vi "repeat cycle_linear up.vi"(8 "error in (no error)":errorcluster caption="에러 입력(에러 없음)", 10 "waveform in":waveform(dbl), 11 "Waveform Obj 입력":refnum<class "PWL_DW7802.lvclass">) -> (0 "error out":errorcluster caption="에러 출력", 2 "waveform out":waveform(dbl), 3 "Waveform Obj 출력":refnum<class "PWL_DW7802.lvclass">)   [LabVIEW 2020, in "PWL_DW7802.lvclass"]
uses:
  PWL_DW7802.lvclass
  Waveform Gen/Waveform Gen.lvclass/Waveform Gen.ctl
  PWL/PWL.lvclass/PWL.ctl
  Waveform Gen/Accessors/Read cycle.vi
  Waveform Gen/Accessors/Read scale.vi
  PWL/Accessors/Read previous pwl scale.vi
  <vilib>/Waveform/WDTOps.llb/WDT Number of Waveform Samples DBL.vi
  <vilib>/Waveform/WDTOps.llb/WDT Get Waveform Subset DBL.vi
  <vilib>/Waveform/WDTOps.llb/WDT Append Waveforms DBL.vi
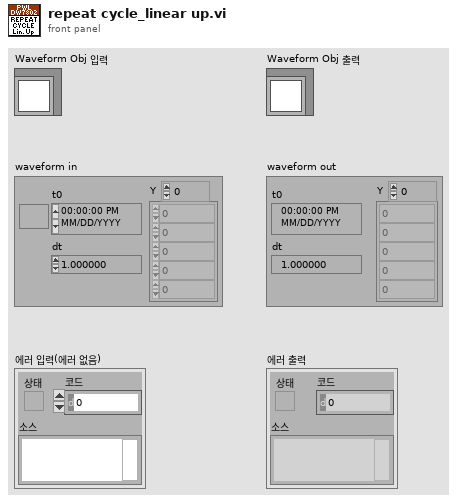
[diagram p1: front panel]
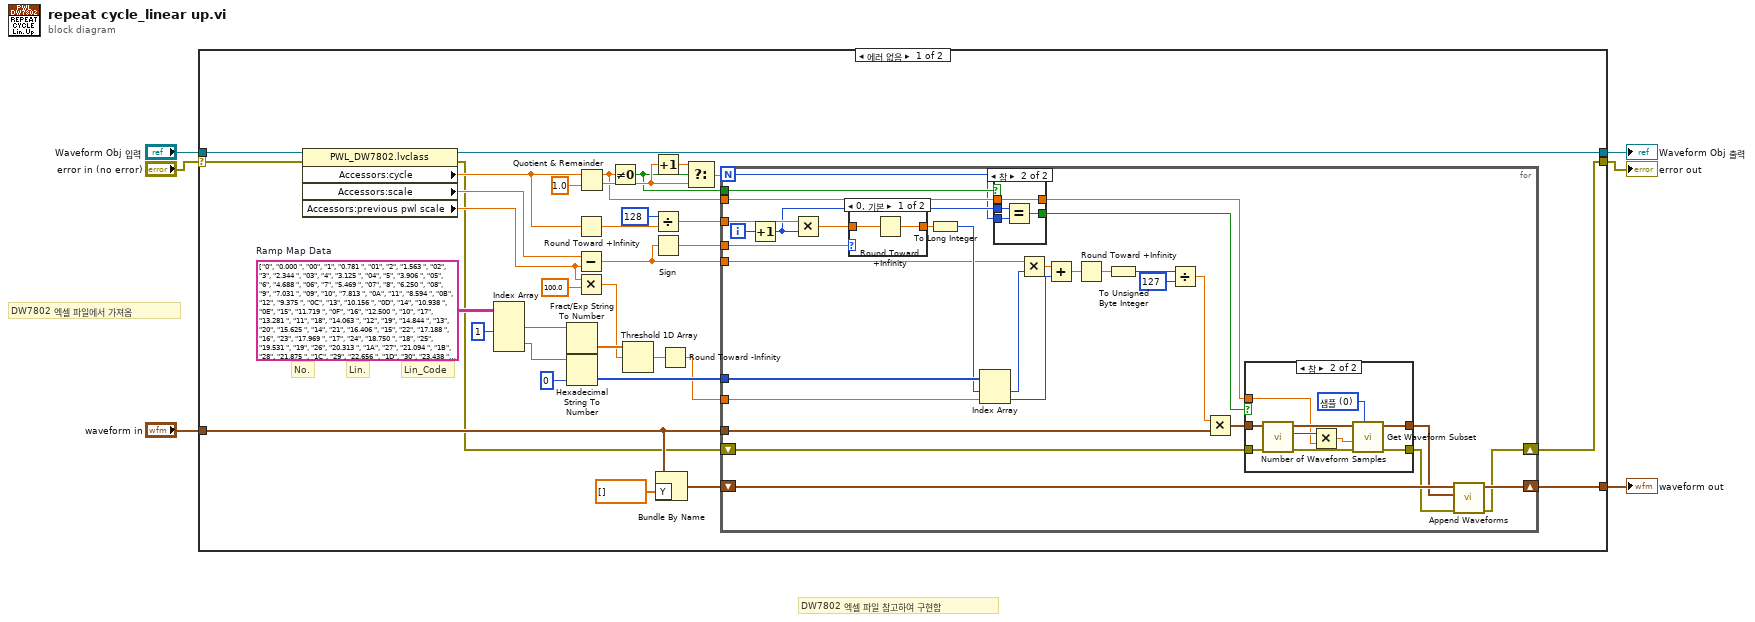
[diagram p0: block diagram]
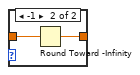
[diagram p2: hidden frame]
diagram:
  # "DW7802 엑셀 파일에서 가져옴"
  # "DW7802 엑셀 파일 참고하여 구현함"
  n1 = case shown="에러 없음" "error in (no error)" {
    selector: "error in (no error)" -> [w39 w92]
    tunnel: "Waveform Obj 입력" -> [w40 w93]
    tunnel: [w38 w93] -> w4
    tunnel: [w15 w92] -> w3
    tunnel: "waveform in" -> [w22 _]
    tunnel: [w14 _] -> w1
    frame No Error {
      w32 = string[][] [["0", "0.000 ", "00"], ["1", "0.781 ", "01"], ["2", "1.563 ", "02"], ["3", "2.344 ", "03"], ["4", "3.125 ", "04"], ["5", "3.906 ", "05"], ["6", "4.688 ", "06"], ["7", "5.469 ", "07"], ["8", "6.250 ", "08"], ["9", "7.031 ", "09"], ["10", "7.813 ", "0A"], ["11", "8.594 ", "0B"], ["12", "9.375 ", "0C"], ["13", "10.156 ", "0D"], ["14", "10.938 ", "0E"], ["15", "11.719 ", "0F"], ["16", "12.500 ", "10"], ["17", "13.281 ", "11"], ["18", "14.063 ", "12"], ["19", "14.844 ", "13"], ["20", "15.625 ", "14"], ["21", "16.406 ", "15"], ["22", "17.188 ", "16"], ["23", "17.969 ", "17"], ["24", "18.750 ", "18"], ["25", "19.531 ", "19"], ["26", "20.313 ", "1A"], ["27", "21.094 ", "1B"], ["28", "21.875 ", "1C"], ["29", "22.656 ", "1D"], ["30", "23.438 ", "1E"], ["31", "24.219 ", "1F"], ["32", "25.000 ", "20"], ["33", "25.781 ", "21"], ["34", "26.563 ", "22"], ["35", "27.344 ", "23"], ["36", "28.125 ", "24"], ["37", "28.906 ", "25"], ["38", "29.688 ", "26"], ["39", "30.469 ", "27"], ["40", "31.250 ", "28"], ["41", "32.031 ", "29"], ["42", "32.813 ", "2A"], ["43", "33.594 ", "2B"], ["44", "34.375 ", "2C"], ["45", "35.156 ", "2D"], ["46", "35.938 ", "2E"], ["47", "36.719 ", "2F"], ["48", "37.500 ", "30"], ["49", "38.281 ", "31"], ["50", "39.063 ", "32"], ["51", "39.844 ", "33"], ["52", "40.625 ", "34"], ["53", "41.406 ", "35"], ["54", "42.188 ", "36"], ["55", "42.969 ", "37"], ["56", "43.750 ", "38"], ["57", "44.531 ", "39"], ["58", "45.313 ", "3A"], ["59", "46.094 ", "3B"], ["60", "46.875 ", "3C"], ["61", "47.656 ", "3D"], ["62", "48.438 ", "3E"], ["63", "49.219 ", "3F"], ["64", "50.000 ", "40"], ["65", "50.781 ", "40"], ["66", "51.563 ", "41"], ["67", "52.344 ", "42"], ["68", "53.125 ", "43"], ["69", "53.906 ", "44"], ["70", "54.688 ", "45"], ["71", "55.469 ", "46"], ["72", "56.250 ", "47"], ["73", "57.031 ", "48"], ["74", "57.813 ", "49"], ["75", "58.594 ", "4A"], ["76", "59.375 ", "4B"], ["77", "60.156 ", "4C"], ["78", "60.938 ", "4D"], ["79", "61.719 ", "4E"], ["80", "62.500 ", "4F"], ["81", "63.281 ", "50"], ["82", "64.063 ", "51"], ["83", "64.844 ", "52"], ["84", "65.625 ", "53"], ["85", "66.406 ", "54"], ["86", "67.188 ", "55"], ["87", "67.969 ", "56"], ["88", "68.750 ", "57"], ["89", "69.531 ", "58"], ["90", "70.313 ", "59"], ["91", "71.094 ", "5A"], ["92", "71.875 ", "5B"], ["93", "72.656 ", "5C"], ["94", "73.438 ", "5D"], ["95", "74.219 ", "5E"], ["96", "75.000 ", "5F"], ["97", "75.781 ", "60"], ["98", "76.563 ", "61"], ["99", "77.344 ", "62"], ["100", "78.125 ", "63"], ["101", "78.906 ", "64"], ["102", "79.688 ", "65"], ["103", "80.469 ", "66"], ["104", "81.250 ", "67"], ["105", "82.031 ", "68"], ["106", "82.813 ", "69"], ["107", "83.594 ", "6A"], ["108", "84.375 ", "6B"], ["109", "85.156 ", "6C"], ["110", "85.938 ", "6D"], ["111", "86.719 ", "6E"], ["112", "87.500 ", "6F"], ["113", "88.281 ", "70"], ["114", "89.063 ", "71"], ["115", "89.844 ", "72"], ["116", "90.625 ", "73"], ["117", "91.406 ", "74"], ["118", "92.188 ", "75"], ["119", "92.969 ", "76"], ["120", "93.750 ", "77"], ["121", "94.531 ", "78"], ["122", "95.313 ", "79"], ["123", "96.094 ", "7A"], ["124", "96.875 ", "7B"], ["125", "97.656 ", "7C"], ["126", "98.438 ", "7D"], ["127", "99.219 ", "7E"], ["128", "100.000 ", "7F"]]  # Ramp Map Data
      # "Lin_Code"
      # "Lin."
      # "No."
      n2 = property class="PWL_DW7802.lvclass"(reference=w40, error in=w39) -> (reference out=w38:refnum<class "PWL_DW7802.lvclass">, error out=w16:errorcluster, "Accessors:cycle"=w26:dbl, "Accessors:scale"=w29:dbl, "Accessors:previous pwl scale"=w28:dbl)
      n3 = Index Array(array=w32, index (col) #1=1 ("비활성화된 인덱스 (열)")) -> (element #1=w37:string[], element #2=w30:string[])  [unwired: 3 in]
      n4 = Fract/Exp String To Number(string=w37) -> (number=w11:dbl[])  [unwired: 3 in, 1 out]
      n5 = Hexadecimal String To Number(string=w30, default (0uL)=u8 0) -> (number=w36:u8[])  [unwired: 1 in, 1 out]
      n6 = Round Toward +Infinity(x=w26) -> (ceil(x): smallest int >= x=w13:dbl)
      n7 = Subtract(x=w29, y=w28) -> (x-y=w8:dbl)
      n8 = Multiply(x=w28, y=100.0) -> (x*y=w10:dbl)
      n9 = Quotient & Remainder(x=w26, y=1.0) -> (x-y*floor(x/y)=w17:dbl, floor(x/y)=w19:dbl)
      n10 = Not Equal To 0?(x=w17) -> (x != 0?=w18:bool)
      n11 = Threshold 1D Array(2:w10, 3:w11) -> (0:w12:dbl)  [unwired: 1 in]
      n12 = Increment(x=w19) -> (x+1=w24:dbl)
      n13 = Divide(x=u8 128 ("y"), y=w13) -> (x/y=w35:dbl)
      n14 = Sign(1:w8) -> (0:w7:dbl)
      n15 = Bundle By Name(cluster=w22, "Y"=dbl[] []) -> (w20:waveform(dbl))
      n16 = Round Toward -Infinity(1:w12) -> (0:w9:dbl)
      n17 = Select(t=w24, s=w18, f=w19) -> (s? t:f=w23:dbl)
      n18 = for {
        N: w23 -> [w51]
        tunnel: w35 -> [w71]
        tunnel: w36 -> [w69]
        tunnel: w8 -> [w64]
        tunnel: w22 -> [w56]
        shift-right: [w46] -> w14
        shift-left: w20 -> [w57]
        tunnel: w18 -> [w54]
        tunnel: w17 -> [w53]
        shift-right: [w43] -> w15
        shift-left: w16 -> [w45]
        tunnel: w9 -> [w42]
        tunnel: w7 -> [w41]
        i -> [w70]
        n19 = Increment(x=w70) -> (x+1=w52:i32)
        n20 = Multiply(x=w71, y=w52) -> (x*y=w68:dbl)
        n21 = case shown="0, 기본" w41 {
          tunnel: w68 -> [w73 w75]
          tunnel: [w72 w74] -> w67
          frame 0, Default {
            n22 = Round Toward +Infinity(x=w73) -> (ceil(x): smallest int >= x=w72:dbl)
          }
          frame -1 {
            n23 = Round Toward -Infinity(1:w75) -> (0:w74:dbl)
          }
        }
        n24 = To Long Integer(number=w67) -> (32bit integer=w66:i32)
        n25 = Index Array(array=w69, index #1=w66, index #2=w42) -> (element #1=w65:u8, element #2=w62:u8)
        n26 = case shown="참" w54 {
          tunnel: w53 -> [_ w89]
          tunnel: w52 -> [_ w91]
          tunnel: w51 -> [_ w90]
          tunnel: [_ w89] -> w49
          tunnel: [_ w88] -> w50
          frame False {
          }
          frame True {
            n27 = Equal?(x=w91, y=w90) -> (x = y?=w88:bool)
          }
        }
        n28 = Multiply(x=w64, y=w65) -> (x*y=w63:dbl)
        n29 = Add(x=w63, y=w62) -> (x+y=w61:dbl)
        n30 = Round Toward +Infinity(x=w61) -> (ceil(x): smallest int >= x=w60:dbl)
        n31 = To Unsigned Byte Integer(number=w60) -> (unsigned 8bit integer=w59:u8)
        n32 = Divide(x=w59, y=u8 127) -> (x/y=w55:dbl)
        n33 = Multiply(x=w55, y=w56) -> (x*y=w48:waveform(dbl))
        n34 = case shown="참" w50 {
          tunnel: w49 -> [_ w81]
          tunnel: w48 -> [w77 w82]
          tunnel: [w77 w80] -> w47
          tunnel: w45 -> [w76 w79]
          tunnel: [w76 w78] -> w44
          frame False {
          }
          frame True {
            w83 = u16 0 items=["샘플", "상대 시간"] ("start/duration format")
            n35 = call-poly <vilib>:"Number of Waveform Samples.vi"("error in (no error)"=w79, "waveform in"=w82) -> ("error out"=w86:errorcluster, "number of samples"=w84:i32, "waveform out"=w87:waveform(dbl))  [unwired: 7 in]
            n36 = Multiply(x=w84, y=w81) -> (x*y=w85:dbl)
            n37 = call-poly <vilib>:"Get Waveform Subset.vi"("start/duration format"=w83, "error in (no error)"=w86, "duration"=w85, "waveform in"=w87) -> ("error out"=w78:errorcluster, "waveform out"=w80:waveform(dbl))  [unwired: 2 in, 2 out]
          }
        }
        n38 = call-poly <vilib>:"Append Waveforms.vi"("error in (no error)"=w44, "waveform B"=w47, "waveform A"=w57) -> ("error out"=w43:errorcluster, "waveform out"=w46:waveform(dbl))  [unwired: 7 in]
      }
    }
    frame Error {
    }
  }
  "error out" <- w3
  "Waveform Obj 출력" <- w4
  "waveform out" <- w1
